vi "Update-buffers.vi"(8 "error in":errorcluster, 11 "Data ref. in":refnum<data-value>) -> (0 "error IO":errorcluster, 3 "Data ref.":refnum<data-value>)   [LabVIEW 2013, in "CameraVision.lvlib" / "CV-Main.lvclass"]
doc: "This function allocates memory resources and creates pointers for temporary processing images, image (batch and queue) buffers and the various characteristics.\nAny old image resources are de-allocated before allocating new ones."
uses:
  CV-Main.lvclass
  CV-Main.lvclass/CV-Main.ctl
  Acquisition/CV-Acquisition.lvclass/CV-Acquisition.ctl
  Configuration/CV-Configuration.lvclass/CV-Configuration.ctl
  Read Buffers.vi
  Read Config params.vi
  Read Acquis params.vi
  Acquisition/Read Batch size var.vi
  Acquisition/Read Image buffer size.vi
  Configuration/Read Number of cameras.vi
  Buffers/CV-Buffers.lvclass
  Configuration/CV-Configuration.lvclass
  Acquisition/CV-Acquisition.lvclass
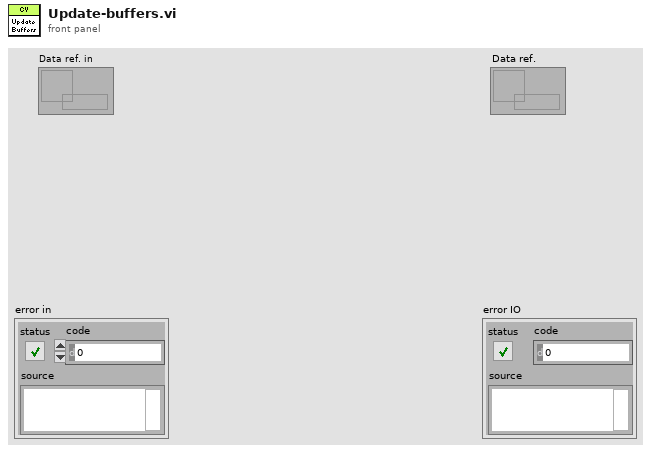
[diagram p1: front panel]
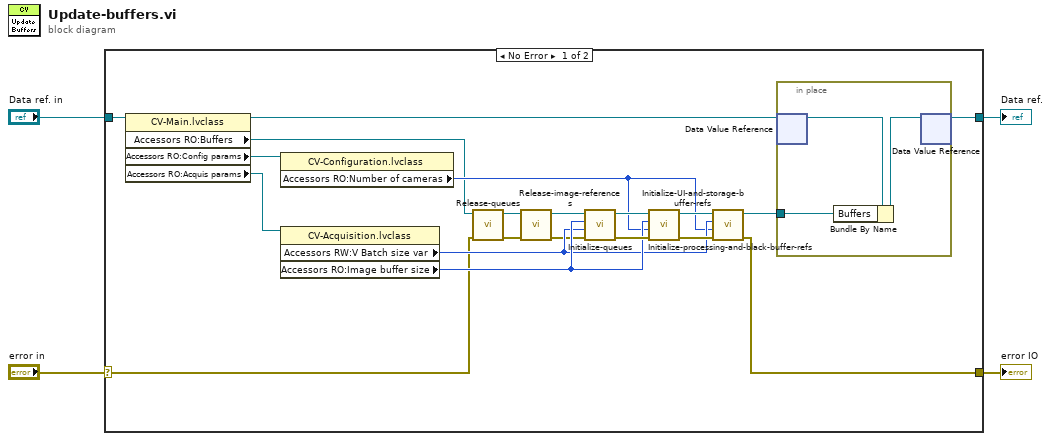
[diagram p0: block diagram]
diagram:
  n1 = case shown="No Error" "error in" {
    selector: "error in" -> [w5 w29]
    tunnel: [w11 w29] -> w4
    tunnel: "Data ref. in" -> [w24 w28]
    tunnel: [w15 w28] -> w1
    frame No Error {
      n2 = property class="CV-Main.lvclass"(reference=w24) -> (reference out=w16:refnum<data-value>, "Accessors RO:Buffers"=w10:refnum<class "CV-Buffers.lvclass">, "Accessors RO:Config params"=w23:refnum<data-value>, "Accessors RO:Acquis params"=w22:refnum<data-value>)  [unwired: 1 in, 1 out]
      n3 = property class="CV-Configuration.lvclass"(reference=w23) -> ("Accessors RO:Number of cameras"=w12:i32)  [unwired: 1 in, 2 out]
      n4 = property class="CV-Acquisition.lvclass"(reference=w22) -> ("Accessors RW:V Batch size var"=w13:i32, "Accessors RO:Image buffer size"=w14:i32)  [unwired: 1 in, 2 out]
      n5 = call "Release-queues.vi"("error in (no error)"=w5, "Buffers in"=w10) -> ("error out"=w9:errorcluster, "Buffers out"=w8:refnum<class "CV-Buffers.lvclass">)  [unwired: 8 in]
      n6 = call "Release-image-references.vi"("error in (no error)"=w9, "Buffers in"=w8) -> ("error out"=w6:errorcluster, "Buffers out"=w7:refnum<class "CV-Buffers.lvclass">)  [unwired: 8 in]
      n7 = call "Initialize-queues.vi"("error in (no error)"=w6, "Batch size"=w13, "Image buffer size"=w14, "Buffers in"=w7) -> ("error out"=w21:errorcluster, "Buffers out"=w19:refnum<class "CV-Buffers.lvclass">)  [unwired: 6 in]
      n8 = call "Initialize-processing-and-black-buffer-refs.vi"("error in (no error)"=w21, "Number of cameras"=w12, "Image buffer size"=w14, "Buffers in"=w19) -> ("error out"=w20:errorcluster, "Buffers out"=w18:refnum<class "CV-Buffers.lvclass">)  [unwired: 6 in]
      n9 = call "Initialize-UI-and-storage-buffer-refs.vi"("error in (no error)"=w20, "Number of cameras"=w12, "Batch size"=w13, "Buffers in"=w18) -> ("error out"=w11:errorcluster, "Buffers out"=w17:refnum<class "CV-Buffers.lvclass">)  [unwired: 6 in]
      n10 = in-place {
        in-place-border: w17 -> [w25]
        n11 = in-place-dvr #1(w16) -> (w27:refnum<class "CV-Main.lvclass">)  [unwired: 1 out]
        n12 = Bundle By Name(cluster=w27, "Buffers"=w25) -> (w26:refnum<class "CV-Main.lvclass">)
        n13 = in-place-dvr #1(w26) -> (w15:refnum<data-value>)  [unwired: 1 out]
      }
    }
    frame Error {
    }
  }
  "error IO" <- w4
  "Data ref." <- w1
